vi "Close.vi"(8 "error in (no error)":errorcluster, 11 "PWM Ref In":T1) -> (0 "error out":errorcluster)   [LabVIEW 2021, in "PWM.lvlib"]
doc: "Closes the reference to a pulse width modulation (PWM) channel. This VI also disables the PWM signal and resets the frequency and duty cycle to zero."
uses:
  <vilib>/myRIO/Instrument Drivers/Onboard IO/PWM/PWM.lvlib
  <vilib>/myRIO/Instrument Drivers/Onboard IO/PWM/typedefs/PWM Reference.ctl
  <vilib>/myRIO/Common/Instrument Driver Framework/Utilities/typedefs/myRIO Generic Hardware Reference.ctl
  <vilib>/myRIO/Common/Instrument Driver Framework/Utilities/typedefs/Hardware Version Enum.ctl
  <vilib>/myRIO/Common/Instrument Driver Framework/Utilities/typedefs/myRIO v1.0 Reference.ctl
  <vilib>/myRIO/Common/Instrument Driver Framework/Utilities/typedefs/Generic FPGA Reference.ctl
  <vilib>/myRIO/Common/Instrument Driver Framework/myRIO v1.0/PWM/typedefs/PWM Channels Enum.ctl
  <vilib>/myRIO/Instrument Drivers/Onboard IO/PWM/typedefs/PWM Configuration.ctl
  <vilib>/myRIO/Common/Instrument Driver Framework/myRIO v1.0/PWM/vis/myRIO v1.0 Unreserve PWM.vi
  <vilib>/myRIO/Common/Instrument Driver Framework/roboRIO v1.0/PWM/vis/roboRIO v1.0 Unreserve PWM.vi
  <vilib>/myRIO/Common/Instrument Driver Framework/myRIO v1.0/PWM/vis/myRIO v1.0 Build MUX Configuration PWM.vi
  <vilib>/myRIO/Common/Instrument Driver Framework/myRIO v1.0/Resource Manager/vis/myRIO v1.0 Unreserve Channel List.vi
  <vilib>/myRIO/Common/Instrument Driver Framework/roboRIO v1.0/Resource Manager/vis/roboRIO v1.0 Unreserve Channel List.vi
  <vilib>/myRIO/Common/Instrument Driver Framework/roboRIO v1.0/PWM/vis/roboRIO v1.0 Build MUX Configuration PWM.vi
  <vilib>/myRIO/Common/Instrument Driver Framework/myRIO v1.0/Resource Manager/vis/myRIO v1.0 Create Configuration List.vi
  <vilib>/myRIO/Common/Instrument Driver Framework/myRIO v1.0/Resource Manager/vis/myRIO v1.0 Unreserve Channel.vi
  <vilib>/myRIO/Common/Instrument Driver Framework/roboRIO v1.0/Resource Manager/vis/roboRIO v1.0 Unreserve Channel.vi
  <vilib>/myRIO/Common/Instrument Driver Framework/roboRIO v1.0/Resource Manager/vis/roboRIO v1.0 Create Configuration List.vi
  <vilib>/myRIO/Common/Instrument Driver Framework/myRIO v1.0/Resource Manager/vis/myRIO v1.0 Build Mutex Name.vi
  <vilib>/myRIO/Common/Instrument Driver Framework/roboRIO v1.0/Resource Manager/vis/roboRIO v1.0 Build Mutex Name.vi
  <vilib>/myRIO/Common/Instrument Driver Framework/myRIO v1.0/PWM/vis/myRIO v1.0 Shutdown PWM.vi
  <vilib>/myRIO/Common/Instrument Driver Framework/myRIO v1.0/Resource Manager/vis/myRIO v1.0 Configure IO.vi
  <vilib>/myRIO/Common/Instrument Driver Framework/Utilities/vis/Configuration Manager.vi
  <vilib>/myRIO/Common/Instrument Driver Framework/Utilities/vis/IO Manager.vi
  <vilib>/myRIO/Common/Instrument Driver Framework/roboRIO v1.0/PWM/vis/roboRIO v1.0 Shutdown PWM.vi
  <vilib>/myRIO/Common/Instrument Driver Framework/roboRIO v1.0/Resource Manager/vis/roboRIO v1.0 Configure IO.vi
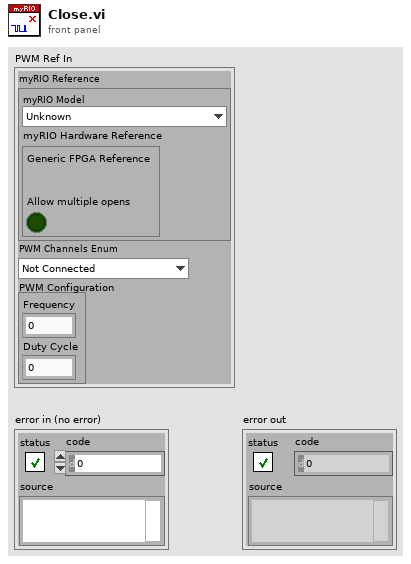
[diagram p1: front panel]
types:
  T1 = typedef "PWM.lvlib/PWM Reference.ctl" = cluster{"myRIO Reference":T2, "PWM Channels Enum":T6, "PWM Configuration":T7}
  T2 = typedef "myRIO Generic Hardware Reference.ctl" = cluster{"myRIO Model":T3, "myRIO Hardware Reference":T4}
  T3 = typedef "Hardware Version Enum.ctl" = enum16{"Unknown", "myRIO-1900", "myRIO-1950", "roboRIO", "NI ELVIS RIO CM", "ELVIS III"}
  T4 = typedef "myRIO v1.0 Reference.ctl" = cluster{"Generic FPGA Reference":T5, "Allow multiple opens":bool}
  T5 = typedef "Generic FPGA Reference.ctl" = refnum<k20>
  T6 = typedef "PWM Channels Enum.ctl" = enum16{"Not Connected", "C/PWM0", "C/PWM1", "A/PWM0", "A/PWM1", "A/PWM2", "A/PWM3", "A/PWM4", "A/PWM5", "A/PWM6", "A/PWM7", "A/PWM8", "A/PWM9", "A/PWM10", "A/PWM11", "A/PWM12", "A/PWM13", "A/PWM14", "A/PWM15", "A/PWM16", "A/PWM17", "A/PWM18", "A/PWM19", "B/PWM0", "B/PWM1", "B/PWM2", "B/PWM3", "B/PWM4", "B/PWM5", "B/PWM6", "B/PWM7", "B/PWM8", "B/PWM9", "B/PWM10", "B/PWM11", "B/PWM12", "B/PWM13", "B/PWM14", "B/PWM15", "B/PWM16", "B/PWM17", "B/PWM18", "B/PWM19", "PWM/PWM0", "PWM/PWM1", "PWM/PWM2", "PWM/PWM3", "PWM/PWM4", "PWM/PWM5", "PWM/PWM6", "PWM/PWM7", "PWM/PWM8", "PWM/PWM9"}
  T7 = typedef "PWM.lvlib/PWM Configuration.ctl" = cluster{"Frequency":dbl, "Duty Cycle":dbl}
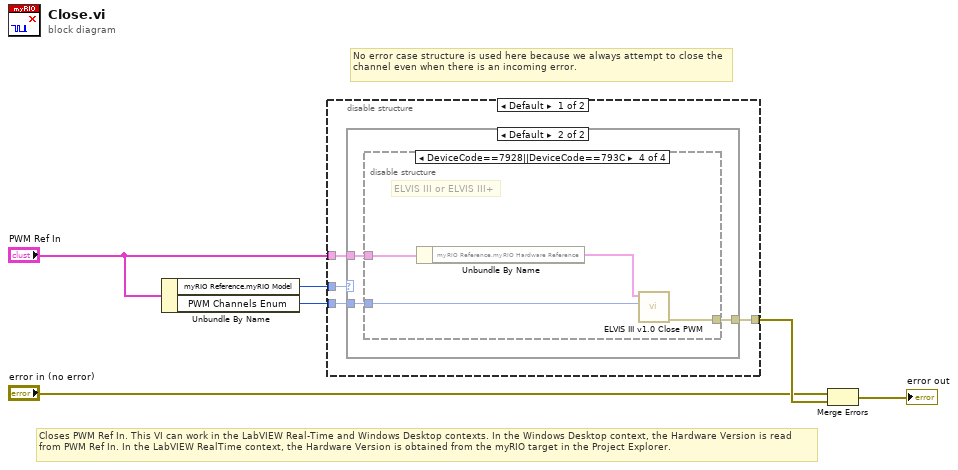
[diagram p0: block diagram]
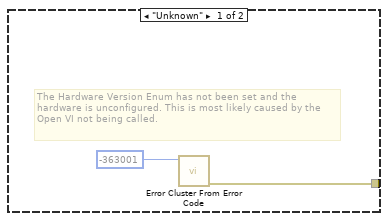
[diagram p2: hidden frame]
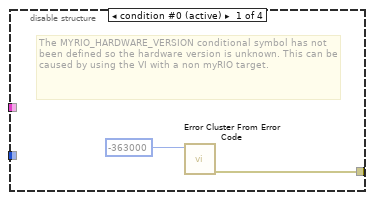
[diagram p3: hidden frame]
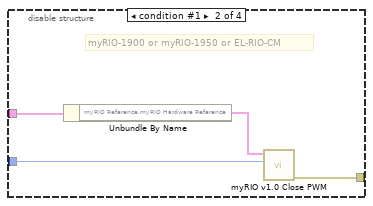
[diagram p4: hidden frame]
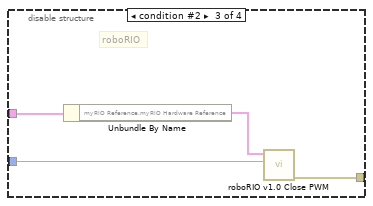
[diagram p5: hidden frame]
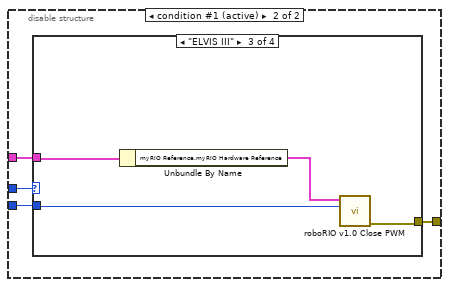
[diagram p6: hidden frame]
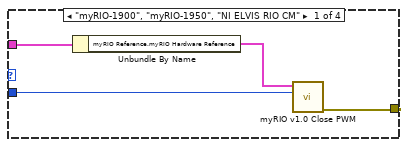
[diagram p7: hidden frame]
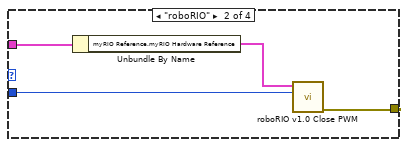
[diagram p8: hidden frame]
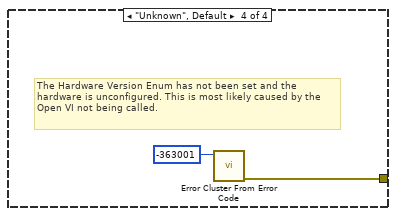
[diagram p9: hidden frame]
diagram:
  # "No error case structure is used here because we always attempt to close the channel even when there is an incoming error."
  # "Closes PWM Ref In. This VI can work in the LabVIEW Real-Time and Windows Desktop contexts. In the Windows Desktop context, the Hardware Version is read from PWM Ref In. In the LabVIEW RealTime context, the Hardware Version is obtained from the myRIO target in the Project Explorer."
  n1 = Unbundle By Name("PWM Ref In") -> ("myRIO Reference.myRIO Model"=w2:T3, "PWM Channels Enum"=w1:T6)
  n2 = disable-structure shown="Default" {
    disable-tunnel: "PWM Ref In" -> [w10 w32]
    disable-tunnel: [w9 w33] -> w6
    disable-tunnel: w2 -> [w8 w31]
    disable-tunnel: w1 -> [w7 w30]
    frame condition #0 {
      n3 = case shown="Default" w8 {
        tunnel: w10 -> [_ w15]
        tunnel: [w11 w14] -> w9
        tunnel: w7 -> [_ w13]
        frame "Unknown" {
          # "The Hardware Version Enum has not been set and the hardware is unconfigured. This is most likely caused by the Open VI not being called."
          n4 = call <vilib>:"Error Cluster From Error Code.vi"("error code (0)"=-363001) -> ("error out"=w11:errorcluster)  [unwired: 8 in]
        }
        frame Default {
          n5 = disable-structure shown="DeviceCode==7928||DeviceCode==793C" {
            disable-tunnel: w15 -> [_ w21 w25 w29]
            disable-tunnel: [w16 w20 w24 w28] -> w14
            disable-tunnel: w13 -> [_ w18 w22 w26]
            frame condition #0 (active) {
              # "The MYRIO_HARDWARE_VERSION conditional symbol has not been defined so the hardware version is unknown. This can be caused by using the VI with a non myRIO target."
              n6 = call <vilib>:"Error Cluster From Error Code.vi"("error code (0)"=-363000) -> ("error out"=w16:errorcluster)  [unwired: 8 in]
            }
            frame condition #1 {
              # "myRIO-1900 or myRIO-1950 or EL-RIO-CM"
              n7 = Unbundle By Name(w21) -> ("myRIO Reference.myRIO Hardware Reference"=w19:T4)
              n8 = call <vilib>:"myRIO v1.0 Close PWM.vi"("PWM Channel"=w18, "myRIO Ref In"=w19) -> ("error out"=w20:errorcluster)  [unwired: 9 in]
            }
            frame condition #2 {
              # "roboRIO"
              n9 = Unbundle By Name(w25) -> ("myRIO Reference.myRIO Hardware Reference"=w23:T4)
              n10 = call <vilib>:"roboRIO v1.0 Close PWM.vi"("PWM Channel"=w22, "myRIO Ref In"=w23) -> ("error out"=w24:errorcluster)  [unwired: 9 in]
            }
            frame condition #3 {
              # "ELVIS III or ELVIS III+"
              n11 = Unbundle By Name(w29) -> ("myRIO Reference.myRIO Hardware Reference"=w27:T4)
              n12 = call <vilib>:"ELVIS III v1.0 Close PWM.vi"("PWM Channel"=w26, "myRIO Ref In"=w27) -> ("error out"=w28:errorcluster)  [unwired: 9 in]
            }
          }
        }
      }
    }
    frame condition #1 (active) {
      n13 = case shown="\"ELVIS III\"" w31 {
        tunnel: w32 -> [w37 w41 w44 _]
        tunnel: [w36 w40 w42 w46] -> w33
        tunnel: w30 -> [w34 w38 w43 _]
        frame "myRIO-1900", "myRIO-1950", "NI ELVIS RIO CM" {
          n14 = Unbundle By Name(w37) -> ("myRIO Reference.myRIO Hardware Reference"=w35:T4)
          n15 = call <vilib>:"myRIO v1.0 Close PWM.vi"("PWM Channel"=w34, "myRIO Ref In"=w35) -> ("error out"=w36:errorcluster)  [unwired: 9 in]
        }
        frame "roboRIO" {
          n16 = Unbundle By Name(w41) -> ("myRIO Reference.myRIO Hardware Reference"=w39:T4)
          n17 = call <vilib>:"roboRIO v1.0 Close PWM.vi"("PWM Channel"=w38, "myRIO Ref In"=w39) -> ("error out"=w40:errorcluster)  [unwired: 9 in]
        }
        frame "ELVIS III" {
          n18 = Unbundle By Name(w44) -> ("myRIO Reference.myRIO Hardware Reference"=w45:T4)
          n19 = call <vilib>:"roboRIO v1.0 Close PWM.vi"("PWM Channel"=w43, "myRIO Ref In"=w45) -> ("error out"=w42:errorcluster)  [unwired: 9 in]
        }
        frame "Unknown", Default {
          # "The Hardware Version Enum has not been set and the hardware is unconfigured. This is most likely caused by the Open VI not being called."
          n20 = call <vilib>:"Error Cluster From Error Code.vi"("error code (0)"=-363001) -> ("error out"=w46:errorcluster)  [unwired: 8 in]
        }
      }
    }
  }
  n21 = Merge Errors("error in (no error)", w6) -> (→"error out":errorcluster)
